vi "DHE_Expose.vi"(2 "error in":errorcluster, 4 "fd":i32) -> (0 "error out":errorcluster)   [LabVIEW 2016]
uses:
  DBSHAND/private/vis/DatabaseHand_Element_Get(bool).vi
  DBSHAND/private/vis/DatabaseHand_Element_Get(string).vi
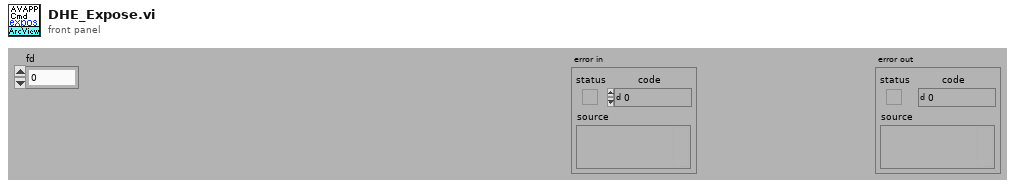
[diagram p1: front panel]
types:
  T1 = typedef "DatabaseHand_RefNum.ctl" = refnum<vi>
  T2 = typedef "DHE_Obs.ctl" = cluster{"observer":string, "obstype":string, "exptime":dbl, "coadds":i32, "fowler":i32, "nimages":i32, "display":bool, "autowrite":bool, "frames to write":cluster{"subs":bool, "reset":bool, "exposed":bool}, "frames to display":cluster{"subs":bool, "reset":bool, "exposed":bool}, "sur":i32}
  T3 = cluster{"Video Processor Type":string, "support gain":bool, "Timing Board":string, "support reset":bool, "Utility Board":string, "Shutter":string, "Temperature":string, "support temp control":bool, "Detector Type":string, "Support MPP":string, "Support Binning":string, "Readout Mode":string, "support shutter control":bool}
  T4 = typedef "CMN_Buffers.ctl" = cluster{"TotalPixels":u32, "Total image bytes":u32, "Total Phys Buffers":u32, "virtual buf pixels":u32, "virtual bytes size":u32, "Remaining piece":u32, "Transfer_Buf_size":u32}
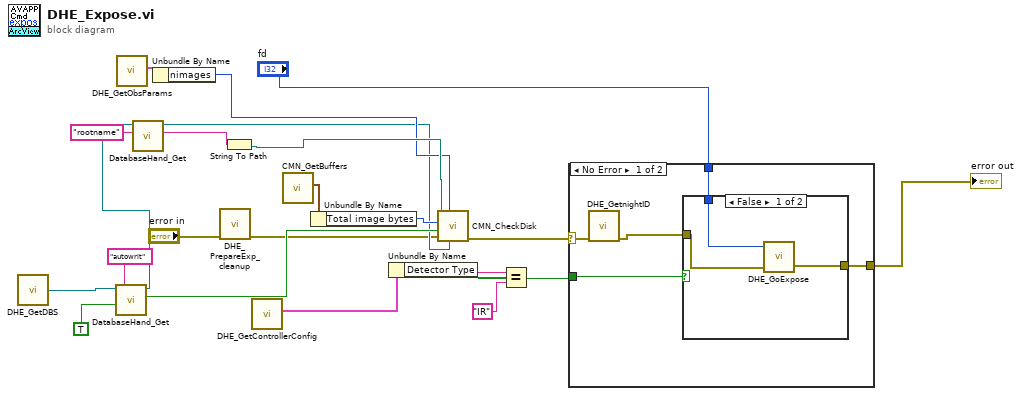
[diagram p0: block diagram]
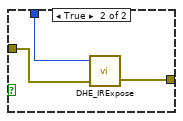
[diagram p2: hidden frame]
diagram:
  n1 = call "DHE_GetDBS.vi"() -> ("DHE_DBSRef"=w7:T1)  [unwired: 9 out]
  n2 = call-poly "DatabaseHand_Get.vi"("default value"=TRUE, "name"="autowrit", "Database RefNum in"=w7) -> ("value"=w13:bool, "Database RefNum out"=w12:T1)  [unwired: 2 in, 5 out]
  n3 = call "DHE_GetObsParams.vi"() -> ("DHE_OBS"=w6:T2)  [unwired: 11 out]
  n4 = call-poly "DatabaseHand_Get.vi"("name"="rootname", "Database RefNum in"=w12) -> ("value"=w10:string, "Database RefNum out"=w4:T1)  [unwired: 3 in, 5 out]
  n5 = Unbundle By Name(w6) -> ("nimages"=w5:i32)
  n6 = call "DHE_PrepareExp_cleanup.vi"("error in (no error)"="error in") -> ("error out"=w1:errorcluster)  [unwired: 10 out]
  n7 = String To Path(string=w10) -> (path=w16:path)
  n8 = call "DHE_GetControllerConfig.vi"() -> ("ControllerConfigCluster"=w17:T3)  [unwired: 11 out]
  n9 = call "CMN_GetBuffers.vi"() -> ("BuffersDimensions"=w8:T4)  [unwired: 2 in, 9 out]
  n10 = Unbundle By Name(w8) -> ("Total image bytes"=w9:u32)
  n11 = Unbundle By Name(w17) -> ("Detector Type"=w20:string)
  n12 = call "CMN_CheckDisk.vi"("DHE_DBSRef"=w4, "num_images (1)"=w5, "error in"=w1, "Generate Error?"=w13, "size in"=w9, "path"=w16) -> ("error out"=w3:errorcluster)  [unwired: 5 out]
  n13 = Equal?(x=w20, y="IR") -> (x = y?=w22:bool)
  n14 = case shown="No Error" w3 {
    selector: w3 -> [w24 w34]
    tunnel: w22 -> [w27 _]
    tunnel: [w26 w34] -> w19
    tunnel: "fd" -> [w25 _]
    frame No Error {
      n15 = call "DHE_GetnightID.vi"("error in (no error)"=w24) -> ("error out"=w23:errorcluster)  [unwired: 10 out]
      n16 = case shown="False" w27 {
        tunnel: w25 -> [w30 w33]
        tunnel: w23 -> [w29 w32]
        tunnel: [w28 w31] -> w26
        frame False {
          n17 = call "DHE_GoExpose.vi"("error in"=w29, "fd"=w30) -> ("error out"=w28:errorcluster)  [unwired: 2 out]
        }
        frame True {
          n18 = call "DHE_IRExpose.vi"("error in"=w32, "fd"=w33) -> ("error out"=w31:errorcluster)  [unwired: 2 out]
        }
      }
    }
    frame Error {
    }
  }
  "error out" <- w19
